vi "Send Ping.vi"(7 "Message Priority (Normal)":T1=enum."Normal", 8 "error in (no error)":errorcluster, 9 "timeout in ms (5000)":i32=5000, 11 "Message Enqueuer":refnum<class "Message Enqueuer.lvclass">) -> (0 "error out":errorcluster, 1 "delay in seconds":dbl, 2 "timed out?":bool, 3 "Message Enqueuer out":refnum<class "Message Enqueuer.lvclass">, 4 "actor quit before receiving ping?":bool)   [LabVIEW 2020, in "Actor Framework.lvlib" / "Ping Msg.lvclass"]
doc: "This VI sends a synchronous message to any actor. This VI outputs the time delay between sending the message and the actor receiving the message (computed using the high-resolution timer). Delay will be zero if there is an error. Errors occur only if the actor has already quit before the ping is sent or if LabVIEW runs out of memory."
uses:
  Ping Msg.lvclass
  Message Enqueuer/Message Enqueuer.lvclass
  C:/justACS/Actor Framework/Core/ActorFramework/Message/Message.lvclass
  C:/justACS/Actor Framework/Core/ActorFramework/tracing/Ping msg/Ping Msg.lvclass
  Message Enqueuer/Message Priority.ctl
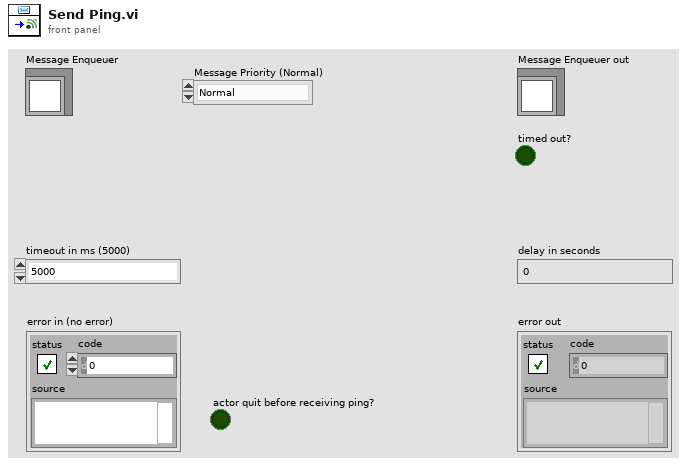
[diagram p1: front panel]
types:
  T1 = typedef "Actor Framework.lvlib/Message Enqueuer.lvclass/Message Priority.ctl" = enum16{"Low", "Normal", "High"}
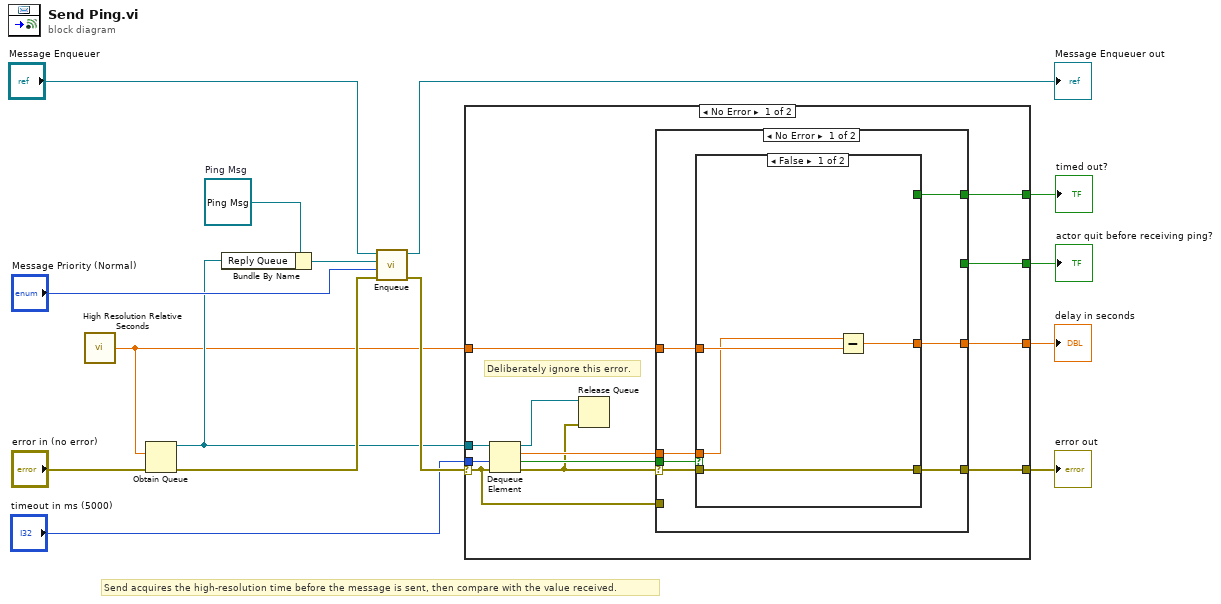
[diagram p0: block diagram]
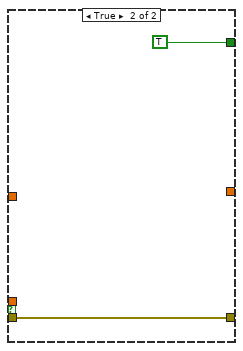
[diagram p2: hidden frame]
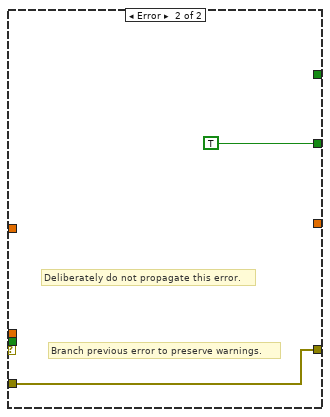
[diagram p3: hidden frame]
diagram:
  w14 = refnum<class "Ping Msg.lvclass"> refnum  # Ping Msg
  # "Send acquires the high-resolution time before the message is sent, then compare with the value received."
  n1 = call <vilib>:"High Resolution Relative Seconds.vi"() -> ("relative seconds"=w3:dbl)
  n2 = Obtain Queue(element data type=w3, error in (no error)="error in (no error)") -> (queue out=w7:refnum<queue>, error out=w9:errorcluster)  [unwired: 3 in, 1 out]
  n3 = Bundle By Name(cluster=w14, "Reply Queue"=w7) -> (w11:refnum<class "Ping Msg.lvclass">)
  n4 = call "Enqueue.vi"("error in (no error)"=w9, "Message Priority (Normal)"="Message Priority (Normal)", "Message"=w11, "Message Enqueuer in"="Message Enqueuer") -> ("error out"=w8:errorcluster, "Message Enqueuer in"=→"Message Enqueuer out":refnum<class "Message Enqueuer.lvclass">)  [unwired: 6 in]
  n5 = case shown="No Error" w8 {
    selector: w8 -> [w16 w43]
    tunnel: w7 -> [w27 _]
    tunnel: "timeout in ms (5000)" -> [w26 _]
    tunnel: [w17 w43] -> w5
    tunnel: [w25 _] -> w4
    tunnel: w3 -> [w24 _]
    tunnel: [w21 _] -> w2
    tunnel: [w20 _] -> w1
    frame No Error {
      # "Deliberately ignore this error."
      n6 = Dequeue Element(queue=w27, timeout in ms (-1)=w26, error in (no error)=w16) -> (queue out=w19:refnum<queue>, element=w23:dbl, timed out?=w22:bool, error out=w18:errorcluster)
      n7 = Release Queue(queue=w19, error in (no error)=w18) -> ()  [unwired: 1 in, 3 out]
      n8 = case shown="No Error" w18 {
        selector: w18 -> [w34 _]
        tunnel: [w33 _] -> w25
        tunnel: w24 -> [w32 _]
        tunnel: w23 -> [w31 _]
        tunnel: w22 -> [w30 _]
        tunnel: [w29 _] -> w21
        tunnel: [_ TRUE] -> w20
        tunnel: [w28 w41] -> w17
        tunnel: w16 -> [_ w41]
        frame No Error {
          n9 = case shown="False" w30 {
            tunnel: w34 -> [w35 w39]
            tunnel: [w38 _] -> w33
            tunnel: w32 -> [w37 _]
            tunnel: w31 -> [w36 _]
            tunnel: [_ TRUE] -> w29
            tunnel: [w35 w39] -> w28
            frame False {
              n10 = Subtract(x=w36, y=w37) -> (x-y=w38:dbl)
            }
            frame True {
            }
          }
        }
        frame Error {
          # "Branch previous error to preserve warnings."
          # "Deliberately do not propagate this error."
        }
      }
    }
    frame Error {
    }
  }
  "error out" <- w5
  "delay in seconds" <- w4
  "timed out?" <- w2
  "actor quit before receiving ping?" <- w1
